vi "Main.vi"() -> ()   [LabVIEW 2017, in "Konfiguracja.lvlib"]
doc: "This template is based from the Queued Message Handler design pattern and the Queued Message Handler Project Template that ships with LabVIEW 2014.\n\nThe main difference is that the Queue is private to this module and communication between modules is done via Broadcast and Request events.\n\nRequest events are wrapped via public API methods and are handled in the Event handler loop in this VI.\nAny module can register for Broadcast events sent by this module.\n\nThe Event Handling Loop generates messages based on user interface actions.\n\nThe Message Handling Loop processes messages generated by the Event Handling Loop, or by other messages. The messages are string values, so new messages can be added easily to the Message Cases case structure in the Message Handling Loop. Each message cluster can also provide an optional value for Message Data, which is a variant that can be converted to whatever message-specific data is required.\n_____\nBased on Delacor QMH Project Template 3.1.0.34."
uses:
  Konfiguracja.lvlib
  <vilib>/Delacor/Delacor QMH/Libraries/Module Admin_class/Delacor_lib_QMH_Module Admin.lvclass
  Module Buttons--radio button.ctl
  Module Data--cluster.ctl
  Show Panel Argument--cluster.ctl
  Hide Panel Argument--cluster.ctl
  Stop Argument--cluster.ctl
  <vilib>/Delacor/Delacor QMH/Libraries/Module Admin_class/Delacor_lib_QMH_Module Admin.lvclass/Delacor_lib_QMH_Module Admin.ctl
  <vilib>/Delacor/Delacor QMH/Libraries/Module Admin_class/Delacor_lib_QMH_Get External Launch.vi
  <vilib>/Utility/error.llb/Error Cluster From Error Code.vi
  <vilib>/Delacor/Delacor QMH/Libraries/Message Queue_class/Delacor_lib_QMH_Enqueue Message (Single).vi
  <vilib>/ErrorRing/Error Ring.xnode
  <vilib>/Delacor/Delacor QMH/Libraries/Message Queue_class/Delacor_lib_QMH_Message Queue.lvclass
panel:
  in  "Select":T1 caption="Radio Buttons"
  out "Logo":bool
  in  "Simulate MHL Error":bool
  in  "Simulate EHL Error":bool
  out "error out":errorcluster
  in  "Module Admin":refnum<class "Delacor_lib_QMH_Module Admin.lvclass">
  out "Status":string
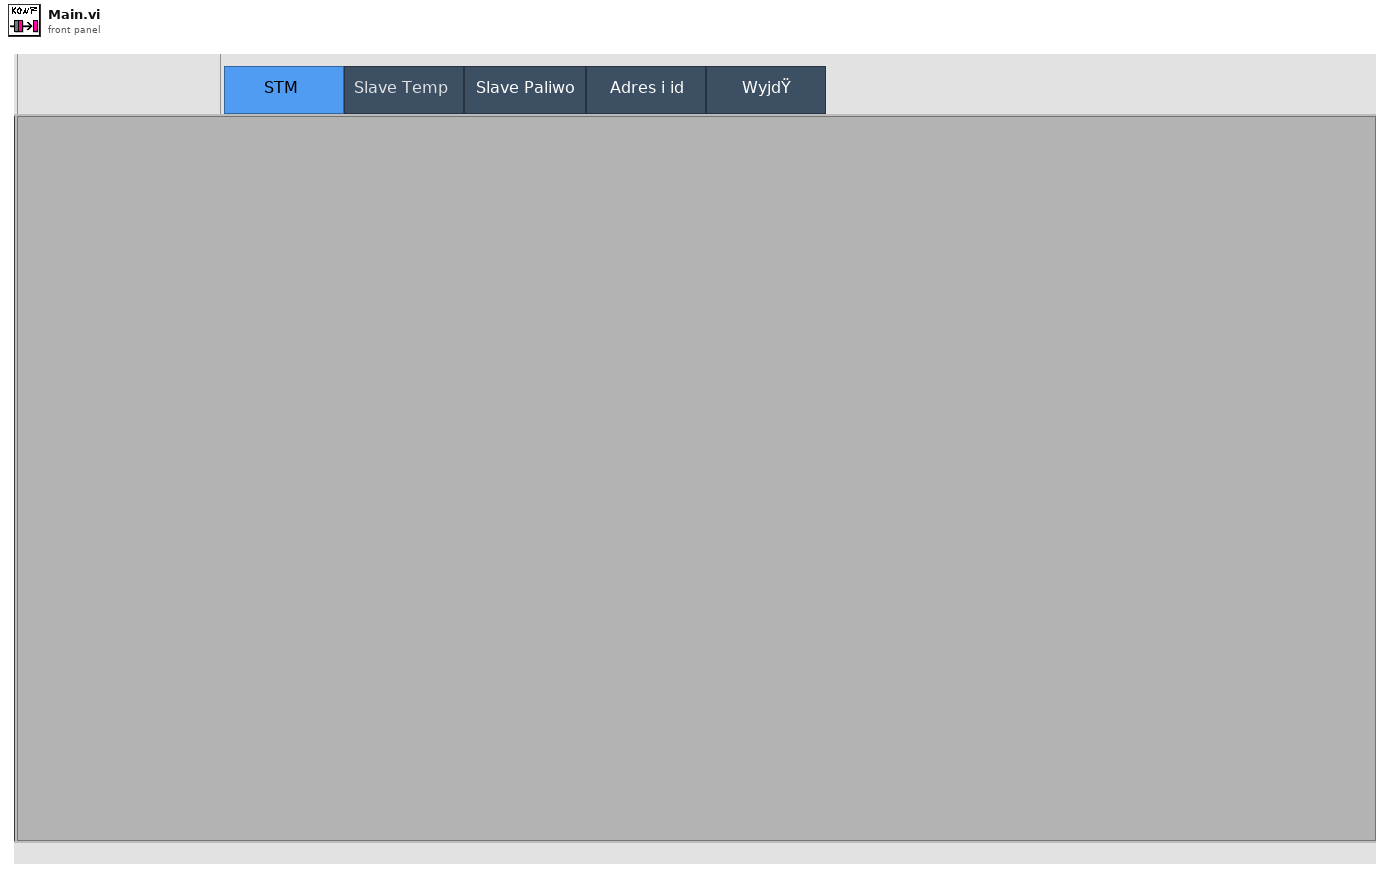
[diagram p1: front panel]
types:
  T1 = typedef "Konfiguracja.lvlib/Module Buttons--radio button.ctl" = enum32{"STM", "Slave_T", "Slave_P", "T_S", "Exit"}
  T2 = typedef "Konfiguracja.lvlib/Request Events--cluster.ctl" = cluster{"Stop Module":refnum<user-event>, "Show Panel":refnum<user-event>, "Hide Panel":refnum<user-event>, "Get Module Execution Status":refnum<user-event>, "Show Diagram":refnum<user-event>}
  T3 = typedef "Konfiguracja.lvlib/Module Data--cluster.ctl" = cluster{"Status":string, "subVI Ref.":refnum<vi>[]}
  T4 = typedef "Konfiguracja.lvlib/Show Panel Argument--cluster.ctl" = cluster{"Show Panel?":bool}
  T5 = typedef "Konfiguracja.lvlib/Hide Panel Argument--cluster.ctl" = cluster{"Hide Panel?":bool}
  T6 = typedef "Konfiguracja.lvlib/Stop Argument--cluster.ctl" = cluster{"Origin":string, "Exit via Stop Module Req?":bool, "Wait for Module to stop?":bool}
  T7 = enum32{"Invalid", "Standard", "Closed", "Hidden", "Minimized", "Maximized"}
  T8 = enum32{"invalid lock state", "Not Locked", "Locked (No Password)", "Password-protected"}
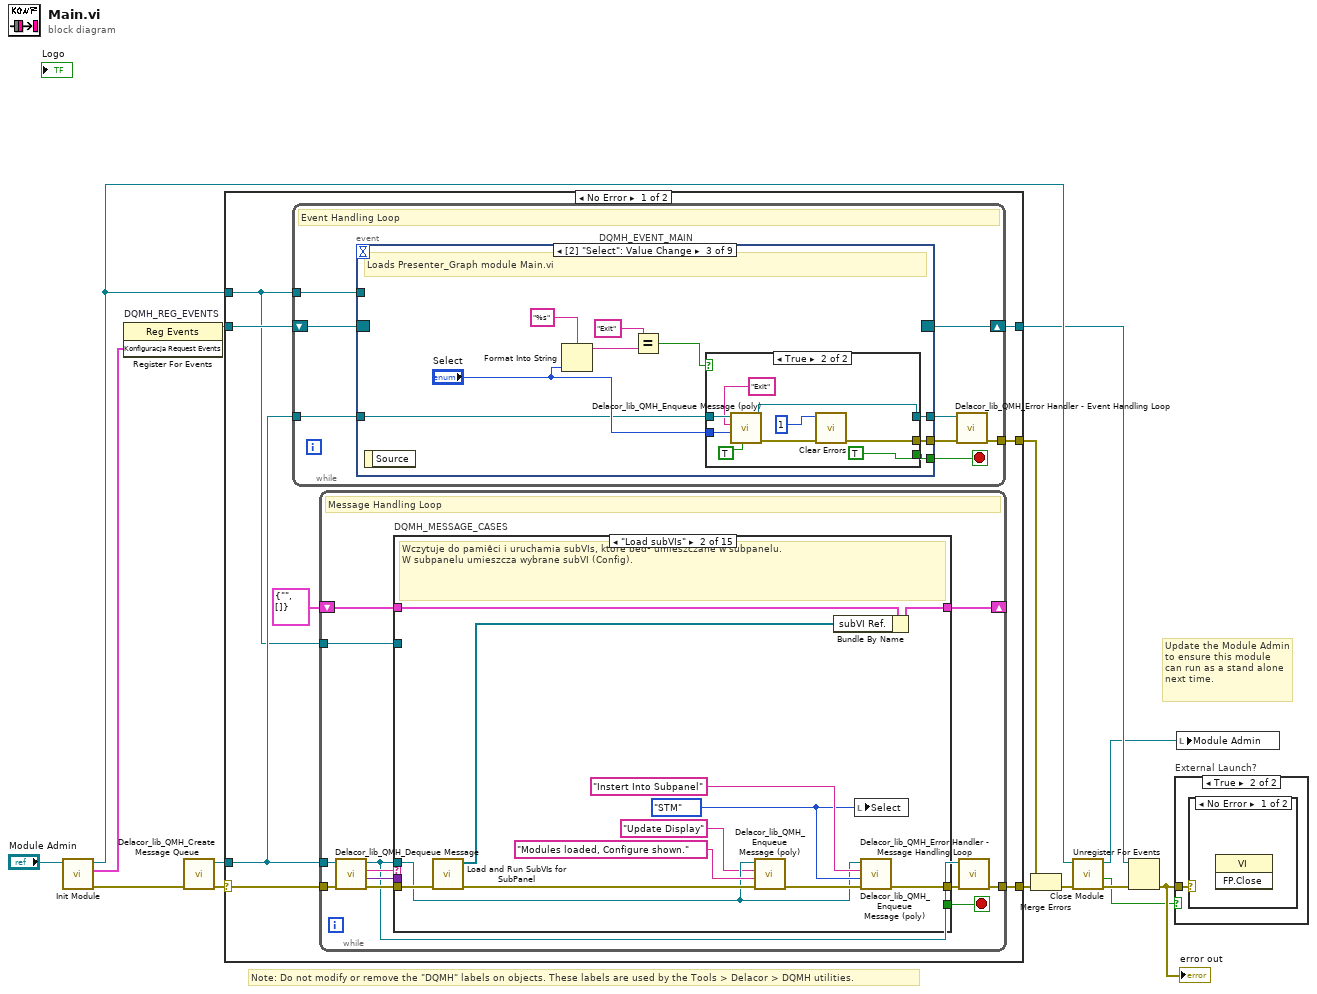
[diagram p0: block diagram]
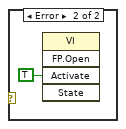
[diagram p3: hidden frame]
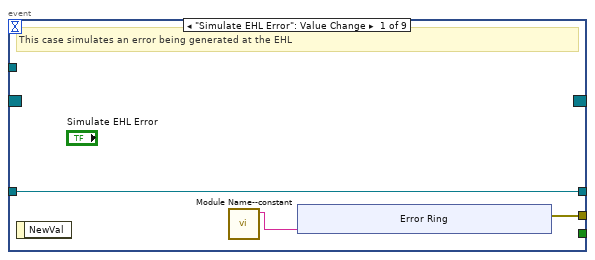
[diagram p4: hidden frame]
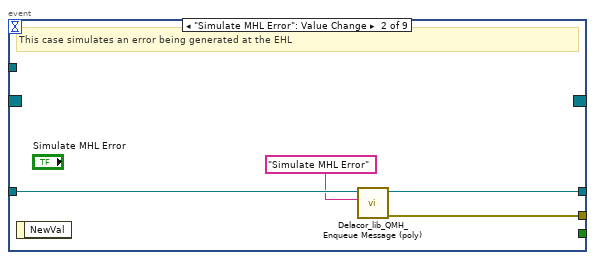
[diagram p5: hidden frame]
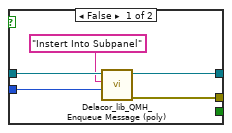
[diagram p6: hidden frame]
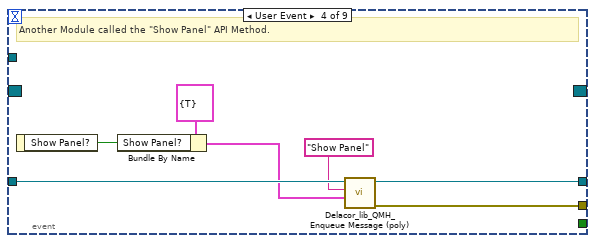
[diagram p7: hidden frame]
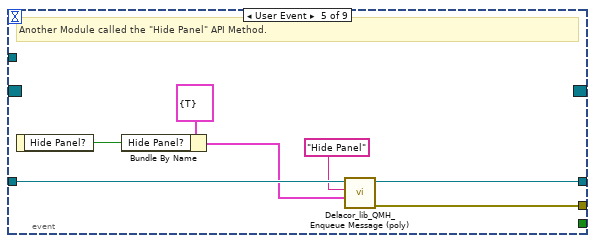
[diagram p8: hidden frame]
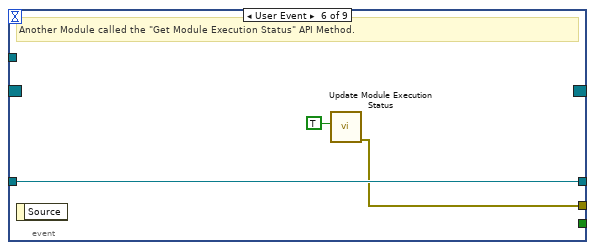
[diagram p9: hidden frame]
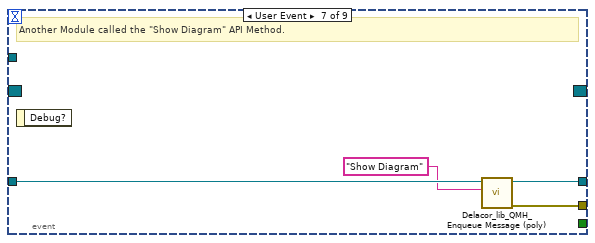
[diagram p10: hidden frame]
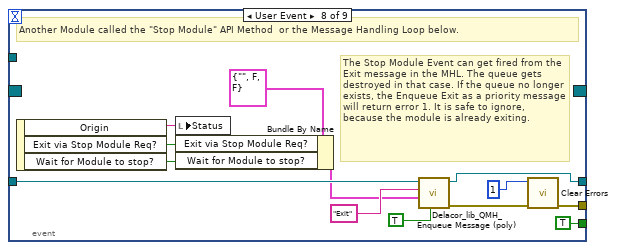
[diagram p11: hidden frame]
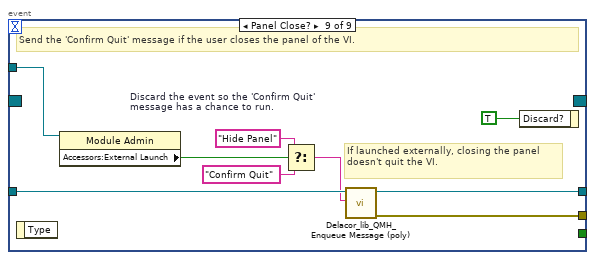
[diagram p12: hidden frame]
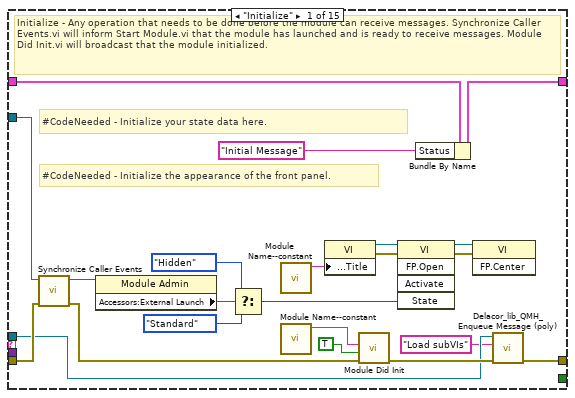
[diagram p13: hidden frame]
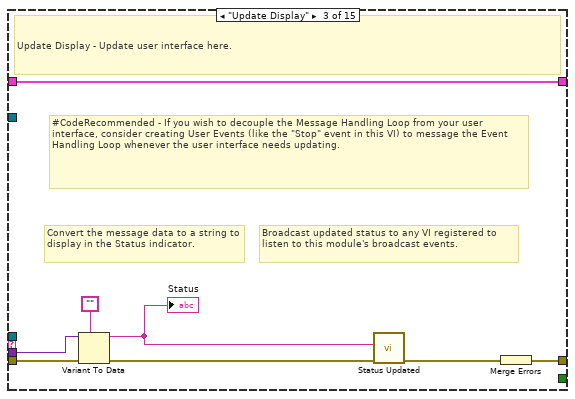
[diagram p14: hidden frame]
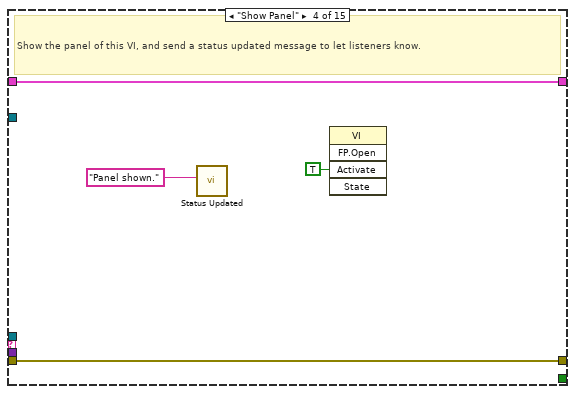
[diagram p15: hidden frame]
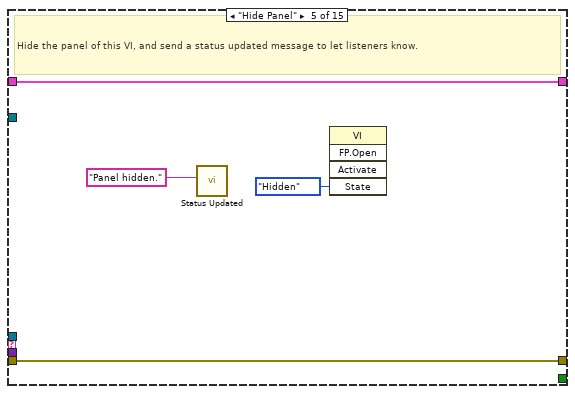
[diagram p16: hidden frame]
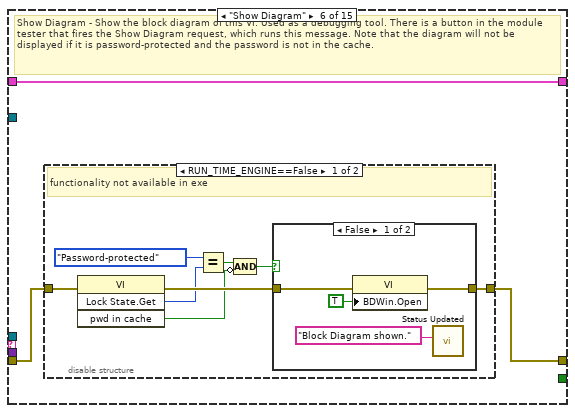
[diagram p17: hidden frame]
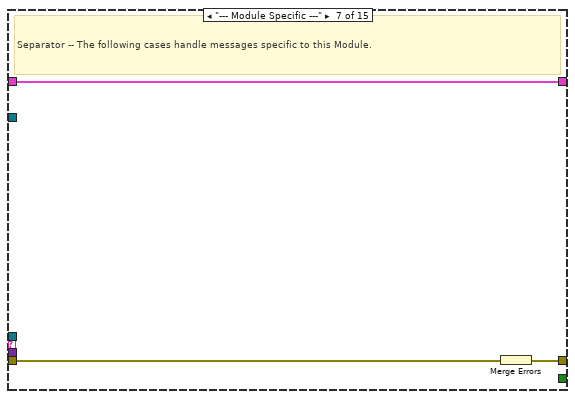
[diagram p20: hidden frame]
diagram:
  # "Note: Do not modify or remove the \"DQMH\" labels on objects. These labels are used by the Tools > Delacor > DQMH utilities."
  # "Update the Module Admin to ensure this module can run as a stand alone next time."
  n1 = call "Init Module.vi"("Singleton Module Admin in"="Module Admin") -> ("error out"=w13:errorcluster, "Konfiguracja Request Events"=w10:T2, "Singleton Module Admin out"=w15:refnum<class "Delacor_lib_QMH_Module Admin.lvclass">)  [unwired: 8 in]
  n2 = register-events "DQMH_REG_EVENTS"(w10) -> (reference out=w11:refnum<event-registration>)  [unwired: 2 in, 1 out]
  n3 = call <vilib>:"Delacor_lib_QMH_Create Message Queue.vi"("error in (no error)"=w13) -> ("error out"=w1:errorcluster, "Message Queue"=w9:refnum<class "Delacor_lib_QMH_Message Queue.lvclass">)  [unwired: 9 in]
  n4 = case shown="No Error" w1 {
    selector: w1 -> [w17 w291]
    tunnel: [w23 w291] -> w14
    tunnel: [w22 w296] -> w12
    tunnel: w11 -> [w20 w296]
    tunnel: w9 -> [w19 _]
    tunnel: [w18 _] -> w5
    tunnel: w15 -> [w16 w292]
    frame No Error {
      n5 = while {
        tunnel: w19 -> [w31]
        shift-right: [w29] -> w22
        shift-left: w20 -> [w30]
        tunnel: [w25] -> w18
        tunnel: w16 -> [w24]
        stop <- w27 stop-if-true
        # "Event Handling Loop"
        n6 = event "DQMH_EVENT_MAIN" shown="[2] \"Select\": Value Change" {
          selector: w30 -> [_ _ _ _ _ _ _ _ _]
          dyn-events: [_ _ _ _ _ _ _ _ _] -> w29
          timeout: _ -> [_ _ _ _ _ _ _ _ _]
          tunnel: [_ _ w46 _ _ _ _ TRUE ("Discard?") _] -> w27
          tunnel: w31 -> [w34 w45 w48 w75 w82 w85 w89 w100 w110]
          tunnel: [w33 w42 w50 w73 w80 w84 w86 w94 w109] -> w28
          tunnel: [w34 w44 w51 w74 w81 w85 w88 w99 w108] -> w26
          tunnel: w24 -> [_ _ _ _ _ _ _ _ w104]
          event "Simulate EHL Error": Value Change {
            # "This case simulates an error being generated at the EHL"
            n7 = event-data() -> ()  [unwired: 1 in, 1 out]
            n8 = call "Module Name--constant.vi"() -> ("Module Name"=w32:string)  [unwired: 11 in]
            n9 = xnode "Error Ring"("parameter 0"=w32) -> ("error out"=w33:errorcluster)
          }
          event "Simulate MHL Error": Value Change {
            # "This case simulates an error being generated at the EHL"
            n10 = event-data() -> ()  [unwired: 1 in, 1 out]
            n11 = call-poly <vilib>:"Delacor_lib_QMH_Enqueue Message (poly).vi"("Message"="Simulate MHL Error", "Message Queue in"=w45) -> ("error out"=w42:errorcluster, "Message Queue out"=w44:refnum<class "Delacor_lib_QMH_Message Queue.lvclass">)  [unwired: 8 in]
          }
          event Value Change {
            # "Loads Presenter_Graph module Main.vi"
            n12 = event-data() -> ()  [unwired: 1 in, 1 out]
            n13 = Format Into String(format string="%s", "Select") -> (resulting string=w53:string)  [unwired: 2 in, 1 out]
            n14 = Equal?(x="Exit", y=w53) -> (x = y?=w47:bool)
            n15 = case shown="True" w47 {
              tunnel: [w59 w68] -> w51
              tunnel: [w58 w61] -> w50
              tunnel: "Select" -> [w57 w67]
              tunnel: w48 -> [w56 w66]
              tunnel: [_ TRUE] -> w46
              frame False {
                n16 = call-poly <vilib>:"Delacor_lib_QMH_Enqueue Message (poly).vi"("Message Data"=w57, "Message"="Instert Into Subpanel", "Message Queue in"=w56) -> ("error out"=w58:errorcluster, "Message Queue out"=w59:refnum<class "Delacor_lib_QMH_Message Queue.lvclass">)  [unwired: 7 in]
              }
              frame True {
                n17 = call-poly <vilib>:"Delacor_lib_QMH_Enqueue Message (poly).vi"("Priority Message? (F)"=TRUE, "Message Data"=w67, "Message"="Exit", "Message Queue in"=w66) -> ("error out"=w62:errorcluster, "Message Queue out"=w68:refnum<class "Delacor_lib_QMH_Message Queue.lvclass">)  [unwired: 6 in]
                n18 = call <vilib>:"Clear Errors.vi"("error in (no error)"=w62, "specific error code to clear (0: all)"=1) -> ("error out"=w61:errorcluster)  [unwired: 4 in, 1 out]
              }
            }
          }
          event User Event {
            # "Another Module called the \"Show Panel\" API Method."
            n19 = event-data() -> ("Show Panel?"=w71:bool)  [unwired: 1 in]
            n20 = Bundle By Name(cluster=T4 {"Show Panel?"=TRUE} ("Show Panel Argument"), "Show Panel?"=w71) -> (w69:T4)
            n21 = call-poly <vilib>:"Delacor_lib_QMH_Enqueue Message (poly).vi"("Message Data"=w69, "Message"="Show Panel", "Message Queue in"=w75) -> ("error out"=w73:errorcluster, "Message Queue out"=w74:refnum<class "Delacor_lib_QMH_Message Queue.lvclass">)  [unwired: 7 in]
          }
          event User Event {
            # "Another Module called the \"Hide Panel\" API Method."
            n22 = event-data() -> ("Hide Panel?"=w77:bool)  [unwired: 1 in]
            n23 = Bundle By Name(cluster=T5 {"Hide Panel?"=TRUE} ("Hide Panel Argument"), "Hide Panel?"=w77) -> (w76:T5)
            n24 = call-poly <vilib>:"Delacor_lib_QMH_Enqueue Message (poly).vi"("Message Data"=w76, "Message"="Hide Panel", "Message Queue in"=w82) -> ("error out"=w80:errorcluster, "Message Queue out"=w81:refnum<class "Delacor_lib_QMH_Message Queue.lvclass">)  [unwired: 7 in]
          }
          event User Event {
            # "Another Module called the \"Get Module Execution Status\" API Method."
            n25 = event-data() -> ()  [unwired: 1 in, 1 out]
            n26 = call "Update Module Execution Status.vi"("Running?"=TRUE) -> ("error out"=w84:errorcluster)  [unwired: 10 in]
          }
          event User Event {
            # "Another Module called the \"Show Diagram\" API Method."
            n27 = event-data() -> ()  [unwired: 1 in, 1 out]
            n28 = call-poly <vilib>:"Delacor_lib_QMH_Enqueue Message (poly).vi"("Message"="Show Diagram", "Message Queue in"=w89) -> ("error out"=w86:errorcluster, "Message Queue out"=w88:refnum<class "Delacor_lib_QMH_Message Queue.lvclass">)  [unwired: 8 in]
          }
          event User Event {
            # "The Stop Module Event can get fired from the Exit message in the MHL. The queue gets destroyed in that case. If the queue no longer exists, the Enqueue Exit as a priority message will return error 1. It is safe to ignore, because the module is already exiting."
            # "Another Module called the \"Stop Module\" API Method  or the Message Handling Loop below."
            n29 = event-data() -> ("Origin"=w98:string, "Exit via Stop Module Req?"=w92:bool, "Wait for Module to stop?"=w91:bool)  [unwired: 1 in]
            n30 = local write "Status"(w98) -> ()
            n31 = Bundle By Name(cluster=T6 {"Origin"="", "Exit via Stop Module Req?"=FALSE, "Wait for Module to stop?"=FALSE} ("Stop Argument"), "Exit via Stop Module Req?"=w92, "Wait for Module to stop?"=w91) -> (w90:T6)
            n32 = call-poly <vilib>:"Delacor_lib_QMH_Enqueue Message (poly).vi"("Priority Message? (F)"=TRUE, "Message Data"=w90, "Message"="Exit", "Message Queue in"=w100) -> ("error out"=w95:errorcluster, "Message Queue out"=w99:refnum<class "Delacor_lib_QMH_Message Queue.lvclass">)  [unwired: 6 in]
            n33 = call <vilib>:"Clear Errors.vi"("error in (no error)"=w95, "specific error code to clear (0: all)"=1) -> ("error out"=w94:errorcluster)  [unwired: 4 in, 1 out]
          }
          event Panel Close? {
            w111 = TRUE  # Discard the event so the 'Confirm Quit' message has a chance to run.
            # "If launched externally, closing the panel doesn't quit the VI."
            # "Send the 'Confirm Quit' message if the user closes the panel of the VI."
            n34 = event-data() -> ()  [unwired: 1 in, 1 out]
            n35 = property class="Module Admin"(reference=w104) -> ("Accessors:External Launch"=w103:bool)  [unwired: 1 in, 2 out]
            n36 = Select(t="Hide Panel" ("Message"), s=w103, f="Confirm Quit" ("Message")) -> (s? t:f=w105:string)
            n37 = call-poly <vilib>:"Delacor_lib_QMH_Enqueue Message (poly).vi"("Message"=w105, "Message Queue in"=w110) -> ("error out"=w109:errorcluster, "Message Queue out"=w108:refnum<class "Delacor_lib_QMH_Message Queue.lvclass">)  [unwired: 8 in]
            n38 = event-data("Discard?"=w111) -> ()  [unwired: 1 in, 1 out]
          }
        }
        n39 = call-dynamic "Delacor_lib_QMH_Error Handler - Event Handling Loop.vi"("error in (no error)"=w28, "Message Queue in"=w26) -> ("dup error in"=w25:errorcluster)  [unwired: 8 in, 1 out]
      }
      n40 = while {
        tunnel: w19 -> [w115]
        shift-right: [w121] -> _
        shift-left: T3 {"Status"="", "subVI Ref."=[]} ("Data Cluster") -> [w122]
        tunnel: w17 -> [w119]
        tunnel: [w113] -> w23
        tunnel: w16 -> [w112]
        stop <- w120 stop-if-true
        # "Message Handling Loop"
        n41 = call-dynamic "Delacor_lib_QMH_Dequeue Message.vi"("error in (no error)"=w119, "Message Queue in"=w115) -> ("error out"=w118:errorcluster, "Message Data"=w116:variant, "Message"=w117:string, "Message Queue out"=w114:refnum<class "Delacor_lib_QMH_Message Queue.lvclass">)  [unwired: 6 in]
        n42 = case "DQMH_MESSAGE_CASES" shown="\"Load subVIs\"" w117 {
          selector: w117 -> [_ _ _ _ _ _ _ _ _ _ _ _ _ _ w278]
          tunnel: w114 -> [w125 w147 _ _ _ _ _ _ w198 _ _ w234 w249 w269 _]
          tunnel: w118 -> [w135 w154 w163 w169 w170 w175 w193 w196 w214 w218 w223 w240 w253 w271 _]
          tunnel: [w126 w152 w164 w169 w170 w174 w191 w194 w215 w216 w221 w231 w251 w266 w279] -> w123
          tunnel: w122 -> [w134 w157 w165 w168 w173 w176 w192 w195 w209 w217 w222 w239 w252 w258 w280]
          tunnel: [w133 w156 w165 w168 w173 w176 w192 w195 w209 w217 w222 w239 w252 w258 w280] -> w121
          tunnel: [_ _ _ _ _ _ _ _ _ _ _ _ _ w268 _] -> w120
          tunnel: w116 -> [_ _ w162 _ _ _ _ _ w212 _ _ w238 _ w265 _]
          tunnel: w112 -> [w136 _ _ _ _ _ _ _ _ _ _ w233 _ w259 _]
          frame "Initialize" {
            # "#CodeNeeded - Initialize the appearance of the front panel."
            # "#CodeNeeded - Initialize your state data here."
            # "Initialize - Any operation that needs to be done before the module can receive messages. Synchronize Caller Events.vi will inform Start Module.vi that the module has launched and is ready to receive messages. Module Did Init.vi will broadcast that the module initialized."
            n43 = call "Synchronize Caller Events.vi"("error in (no error)"=w135, "Singleton Module Admin in"=w136) -> ("error out"=w129:errorcluster, "Singleton Module Admin out"=w128:refnum<class "Delacor_lib_QMH_Module Admin.lvclass">)  [unwired: 8 in]
            n44 = property class="Module Admin"(reference=w128) -> ("Accessors:External Launch"=w140:bool)  [unwired: 1 in, 2 out]
            n45 = Select(t=T7."Hidden" ("State"), s=w140, f=T7."Standard" ("State")) -> (s? t:f=w137:T7)
            n46 = call "Module Name--constant.vi"() -> ("Module Name"=w145:string)  [unwired: 11 in]
            n47 = call "Module Name--constant.vi"() -> ("Module Name"=w130:string)  [unwired: 11 in]
            n48 = property class="VI"("Front Panel.Title"=w145) -> (reference out=w143:refnum<vi>, error out=w144:errorcluster)  [unwired: 2 in]
            n49 = call "Module Did Init.vi"("error in (no error)"=w129, "Initialized?"=TRUE, "Origin"=w130) -> ("error out"=w127:errorcluster)  [unwired: 8 in]
            n50 = invoke class="VI" method="FP.Open"(reference=w143, error in=w144, "State"=w137) -> (reference out=w142:refnum<vi>, error out=w141:errorcluster)  [unwired: 2 in, 3 out]
            n51 = Bundle By Name(cluster=w134, "Status"="Initial Message" ("Initial Message")) -> (w133:T3)
            n52 = invoke class="VI" method="FP.Center"(reference=w142, error in=w141) -> ()  [unwired: 1 in, 3 out]
            n53 = call-poly <vilib>:"Delacor_lib_QMH_Enqueue Message (poly).vi"("error in (no error)"=w127, "Message"="Load subVIs", "Message Queue in"=w125) -> ("error out"=w126:errorcluster)  [unwired: 7 in, 1 out]
          }
          frame "Load subVIs" {
            w151 = Module_Buttons--radio_button."STM" ("Select")
            # "Wczytuje do pamiêci i uruchamia subVIs, które bêd¹ umieszczane w subpanelu.\nW subpanelu umieszcza wybrane subVI (Config)."
            n54 = call "Load and Run SubVIs for SubPanel.vi"("error in (no error)"=w154) -> ("error out"=w150:errorcluster, "subVIs Ref."=w155:refnum<vi>[])  [unwired: 9 in]
            n55 = call-poly <vilib>:"Delacor_lib_QMH_Enqueue Message (poly).vi"("error in (no error)"=w150, "Message Data"="Modules loaded, Configure shown." ("Message"), "Message"="Update Display", "Message Queue in"=w147) -> ("error out"=w149:errorcluster)  [unwired: 6 in, 1 out]
            n56 = Bundle By Name(cluster=w157, "subVI Ref."=w155) -> (w156:T3)
            n57 = local write "Select"(w151) -> ()
            n58 = call-poly <vilib>:"Delacor_lib_QMH_Enqueue Message (poly).vi"("error in (no error)"=w149, "Message Data"=w151, "Message"="Instert Into Subpanel", "Message Queue in"=w147) -> ("error out"=w152:errorcluster)  [unwired: 6 in, 1 out]
          }
          frame "Update Display" {
            # "Broadcast updated status to any VI registered to listen to this module's broadcast events."
            # "Convert the message data to a string to display in the Status indicator."
            # "#CodeRecommended - If you wish to decouple the Message Handling Loop from your user interface, consider creating User Events (like the \"Stop\" event in this VI) to message the Event Handling Loop whenever the user interface needs updating."
            # "Update Display - Update user interface here."
            n59 = Variant To Data(error in=w163, type="", Variant=w162) -> (data=w160:string, error out=w159:errorcluster)
            "Status" <- w160
            n60 = call "Status Updated.vi"("error in (no error)"=w159, "Status"=w160) -> ("error out"=w158:errorcluster)  [unwired: 9 in]
            n61 = Merge Errors(w158) -> (w164:errorcluster)
          }
          frame "Show Panel" {
            # "Show the panel of this VI, and send a status updated message to let listeners know."
            n62 = call "Status Updated.vi"("Status"="Panel shown." ("format string")) -> ()  [unwired: 10 in, 1 out]
            n63 = invoke class="VI" method="FP.Open"("Activate"=TRUE ("Activate?")) -> ()  [unwired: 4 in, 5 out]
          }
          frame "Hide Panel" {
            # "Hide the panel of this VI, and send a status updated message to let listeners know."
            n64 = call "Status Updated.vi"("Status"="Panel hidden." ("format string")) -> ()  [unwired: 10 in, 1 out]
            n65 = invoke class="VI" method="FP.Open"("State"=T7."Hidden") -> ()  [unwired: 4 in, 5 out]
          }
          frame "Show Diagram" {
            # "Show Diagram - Show the block diagram of this VI. Used as a debugging tool. There is a button in the module tester that fires the Show Diagram request, which runs this message. Note that the diagram will not be displayed if it is password-protected and the password is not in the cache."
            n66 = disable-structure shown="RUN_TIME_ENGINE==False" {
              disable-tunnel: [w184 w190] -> w174
              disable-tunnel: w175 -> [w183 w190]
              frame condition #0 (active) {
                # "functionality not available in exe"
                n67 = invoke class="VI" method="Lock State.Get"(error in=w183) -> (error out=w182:errorcluster, "Get Lock State"=w181:T8, "pwd in cache"=w178:bool)  [unwired: 3 in, 1 out]
                n68 = Equal?(x=T8."Password-protected", y=w181) -> (x = y?=w179:bool)
                n69 = Compound Arithmetic op=AND(w179, invert w178) -> (w177:bool)
                n70 = case shown="False" w177 {
                  tunnel: [w187 w189] -> w184
                  tunnel: w182 -> [w185 w189]
                  frame False {
                    n71 = property class="VI"(error in=w185, "BDWin.Open"=TRUE ("Block Diagram Window:Open")) -> (error out=w187:errorcluster)  [unwired: 1 in, 1 out]
                    n72 = call "Status Updated.vi"("Status"="Block Diagram shown." ("format string")) -> ()  [unwired: 10 in, 1 out]
                  }
                  frame True {
                    # "Password-protected VI, and the password is not in the cache. Do not show the diagram."
                  }
                }
              }
              frame condition #1 {
              }
            }
          }
          frame "--- Module Specific ---" {
            # "Separator -- The following cases handle messages specific to this Module."
            n73 = Merge Errors(w193) -> (w191:errorcluster)
          }
          frame "---Copy This Frame---" {
            # "Duplicate this frame when creating new messages.  Change this comment in the duplicated frame to describe this message."
            n74 = Merge Errors(w196) -> (w194:errorcluster)
          }
          frame "Instert Into Subpanel" {
            # "Instert VI into subpanel"
            n75 = Unbundle By Name(w209) -> ("subVI Ref."=w208:refnum<vi>[])
            n76 = Variant To Data(error in=w214, type=Module_Buttons--radio_button."STM" ("Select"), Variant=w212) -> (data=w207:T1, error out=w211:errorcluster)
            n77 = Index Array(array=w208, index=w207) -> (element=w206:refnum<vi>)
            n78 = invoke on="Sub Panel" class="SubPnl" method="Remove VI"(error in=w211) -> (error out=w210:errorcluster)  [unwired: 2 in, 2 out]
            n79 = invoke on="Sub Panel" class="SubPnl" method="Insert VI"(error in=w210, "VI Ref"=w206) -> (error out=w213:errorcluster)  [unwired: 2 in, 3 out]
            n80 = property class="VI"(reference=w206) -> ("Name"=w202:string, "Front Panel.Title"=w197:string)  [unwired: 1 in, 2 out]
            n81 = Concatenate Strings(w197, " loaded" ("string")) -> (w200:string)
            n82 = call "Subpanel VI Loaded.vi"("error in (no error)"=w213, "VI Name"=w202) -> ("error out"=w204:errorcluster)  [unwired: 9 in]
            n83 = call-poly <vilib>:"Delacor_lib_QMH_Enqueue Message (poly).vi"("error in (no error)"=w204, "Message Data"=w200, "Message"="Update Display", "Message Queue in"=w198) -> ("error out"=w203:errorcluster)  [unwired: 6 in, 1 out]
            n84 = Merge Errors(w203) -> (w215:errorcluster)
          }
          frame "--- Exit and Error Handling---" {
            # "Separator - The following cases handle errors and exit messages."
            n85 = Merge Errors(w218) -> (w216:errorcluster)
          }
          frame "Simulate MHL Error" {
            # "Simulate an error occurring at the MHL"
            n86 = call "Module Name--constant.vi"() -> ("Module Name"=w220:string)  [unwired: 11 in]
            n87 = xnode "Error Ring"("parameter 0"=w220) -> ("error out"=w219:errorcluster)
            n88 = Merge Errors(w223, w219) -> (w221:errorcluster)
          }
          frame "Error" {
            # "#CodeRecommended - If you ever change the name of this \"Error\" message, you'll need to update the name in the Check Loop Error.vi as well."
            # "#CodeRecommended - If the module is running in standalone mode (External Launch = FALSE), this code will pop up an error dialog and call the 'Exit' message if an error occurs. Add more fine-grained error handling here."
            # "Error - Check the error message data and respond accordingly. This message is sent by the \"Error Handler\" VIs at the end of each loop in this application."
            n89 = property class="Module Admin"(reference=w233) -> ("Accessors:External Launch"=w232:bool)  [unwired: 1 in, 2 out]
            n90 = Variant To Data(error in=w240, type=errorcluster {"status"=FALSE, "code"=0, "source"=""} ("error constant"), Variant=w238) -> (data=w241:errorcluster, error out=w236:errorcluster)
            n91 = call "Error Reported.vi"("Error"=w241) -> ()  [unwired: 10 in, 1 out]
            n92 = case shown="False" w232 {
              tunnel: [w246 _] -> w235
              tunnel: w234 -> [w245 _]
              tunnel: w241 -> [w242 _]
              frame False {
                # "If the module is running standalone, then pop up an error dialog and call the \"Exit\" message."
                n93 = call <vilib>:"Simple Error Handler.vi"("error in (no error)"=w242) -> ()  [unwired: 4 in, 5 out]
                n94 = call-poly <vilib>:"Delacor_lib_QMH_Enqueue Message (poly).vi"("Priority Message? (F)"=TRUE, "Message"="Exit", "Message Queue in"=w245) -> ("error out"=w246:errorcluster)  [unwired: 7 in, 1 out]
              }
              frame True {
                # "If the module was launched externally, calling the Error Reported broadcast VI is the only action performed by the \"Error\" message. The module's caller can then process the error appropriately."
              }
            }
            n95 = Merge Errors(w236, w235) -> (w231:errorcluster)
            n96 = local write "error out"(w231) -> ()
          }
          frame "Confirm Quit" {
            # "#CodeNeeded - If you want to provide an \"Are you sure\" dialog (or some other notification) before the application exits, place that code here. This message is typically sent from a Panel Close? event."
            # "Confirm Quit - Message that can confirm whether or not the user wants to exit the application."
            n97 = call-poly <vilib>:"Delacor_lib_QMH_Enqueue Message (poly).vi"("Priority Message? (F)"=TRUE, "error in (no error)"=w253, "Message"="Exit", "Message Queue in"=w249) -> ("error out"=w250:errorcluster)  [unwired: 6 in, 1 out]
            n98 = Merge Errors(w250) -> (w251:errorcluster)
          }
          frame "Exit" {
            w263 = 91  # 91: not all Exit messages will have an argument
            w268 = TRUE  # Stop the VI
            # "#CodeNeeded: In most applications, a more sophisticated communication mechanism between the main VI and the plugin VIs should be used in favor of aborting plugin VIs."
            # "Release the message queue reference"
            # "#CodeNeeded - Add any required cleanup code here"
            # "Exit - Exit the application."
            n99 = control-ref of="This VI"() -> (w260:refnum<vi>)
            n100 = Variant To Data(error in=w271, type=T6 {"Origin"="", "Exit via Stop Module Req?"=FALSE, "Wait for Module to stop?"=FALSE} ("Stop Argument"), Variant=w265) -> (data=w261:T6, error out=w264:errorcluster)
            n101 = call "Handle Exit.vi"("Stop Argument"=w261, "Admin in"=w259, "VI reference"=w260) -> ("error out"=w257:errorcluster)  [unwired: 7 in, 1 out]
            n102 = call <vilib>:"Clear Errors.vi"("error in (no error)"=w264, "specific error code to clear (0: all)"=w263) -> ("error out"=w270:errorcluster)  [unwired: 4 in, 1 out]
            n103 = Unbundle By Name(w258) -> ("subVI Ref."=w254:refnum<vi>[])
            n104 = invoke on="Sub Panel" class="SubPnl" method="Remove VI"(error in=w257) -> (error out=w255:errorcluster)  [unwired: 2 in, 2 out]
            n105 = for {
              shift-right: [w276] -> w256
              shift-left: w255 -> [w275]
              tunnel: w254 -> [w272] mode=indexing
              n106 = invoke class="VI" method="Abort VI"(reference=w272, error in=w275) -> (reference out=w273:refnum<vi>, error out=w274:errorcluster)  [unwired: 1 in, 1 out]
              n107 = Close Reference(reference=w273, error in (no error)=w274) -> (error out=w276:errorcluster)
            }
            n108 = call-dynamic "Delacor_lib_QMH_Release Message Queue.vi"("error in (no error)"=w270, "Message Queue"=w269) -> ("error out"=w267:errorcluster)  [unwired: 9 in]
            n109 = Merge Errors(w256, w267) -> (w266:errorcluster)
          }
          frame Default {
            # "'Default' case only runs if there is a message that isn't defined in any of the other cases.  Output a programming error."
            n110 = call "Module Name--constant.vi"() -> ("Module Name"=w277:string)  [unwired: 11 in]
            n111 = xnode "Error Ring"("parameter 0"=w278, "parameter 1"=w277) -> ("error out"=w279:errorcluster)
          }
        }
        n112 = call-dynamic "Delacor_lib_QMH_Error Handler - Message Handling Loop.vi"("error in (no error)"=w123, "Message Queue in"=w114) -> ("dup error in"=w113:errorcluster)  [unwired: 8 in, 1 out]
      }
    }
    frame Error {
      # "Synchronize Caller Events.vi will inform Start Module.vi that the module has launched and will let the code calling Start Module.vi register for broadcasts and would permit the caller receive the broadcast that an error occurred at launch time."
      n113 = call "Synchronize Caller Events.vi"("Singleton Module Admin in"=w292) -> ("error out"=w289:errorcluster)  [unwired: 9 in, 1 out]
      n114 = call "Module Name--constant.vi"() -> ("Module Name"=w295:string)  [unwired: 11 in]
      n115 = Format Into String(format string="An error occurred during initialization. %s is no longer running.", w295) -> (resulting string=w293:string)  [unwired: 2 in, 1 out]
      n116 = Merge Errors(w291, w289) -> (w290:errorcluster)
      n117 = call "Error Reported.vi"("Additional Information"=w293, "Error"=w290) -> ()  [unwired: 9 in, 1 out]
    }
  }
  n118 = Merge Errors(w5, w14) -> (w4:errorcluster)
  n119 = call "Close Module.vi"("error in (no error)"=w4, "Module Admin in"=w15) -> ("error out"=w7:errorcluster, "External Launch"=w2:bool, "Module Admin out"=w6:refnum<class "Delacor_lib_QMH_Module Admin.lvclass">)  [unwired: 7 in]
  n120 = Unregister For Events(event registration refnum=w12, error in=w7) -> (error out=w3:errorcluster)
  "error out" <- w3
  n121 = case "External Launch?" shown="True" w2 {
    tunnel: w3 -> [_ w297]
    frame False {
    }
    frame True {
      n122 = case shown="No Error" w297 {
        frame No Error {
          n123 = invoke class="VI" method="FP.Close"() -> ()  [unwired: 3 in, 3 out]
        }
        frame Error {
          n124 = invoke class="VI" method="FP.Open"("Activate"=TRUE ("Activate?")) -> ()  [unwired: 4 in, 5 out]
        }
      }
    }
  }
  n125 = local write "Module Admin"(w6) -> ()
